vi "Mover4_Control_Forward_Kinematics_Stream_Connection.vi"() -> ()   [LabVIEW 2015]
uses:
  <vilib>/silver_ctls/ArrayMatrixCluster/Real Matrix NI_Silver.ctl
  <vilib>/Utility/miscctls.llb/LVRGBAColorTypeDef.ctl
  <vilib>/robotics/Kinematics/Robot/Forward Kinematics (Point).vi
  <vilib>/robotics/Kinematics/NI_Kinematics.lvlib
  <vilib>/robotics/Kinematics/Plotting/NI_Robotics_3DKinematics.lvlib
panel:
  out "Motor positions (degree)":T1(array[cluster]) {"Error Code (bits)" format="%b"}
  out "End effector transform":T2 format="%#_3g"
  in  "Reset To Zero?":bool
  out "Simulation":refnum<vi>(3d-picture)
  in  "Angles (degree)":dbl[](array[numeric])
  in  "Target IP Address":string="172.22.11.2"
  in  "Stop":bool
  # "In the last column you can see the end effector coordinates (according\nto the theory). This way, you can verify if the real robot reaches this position\ncorrectly."
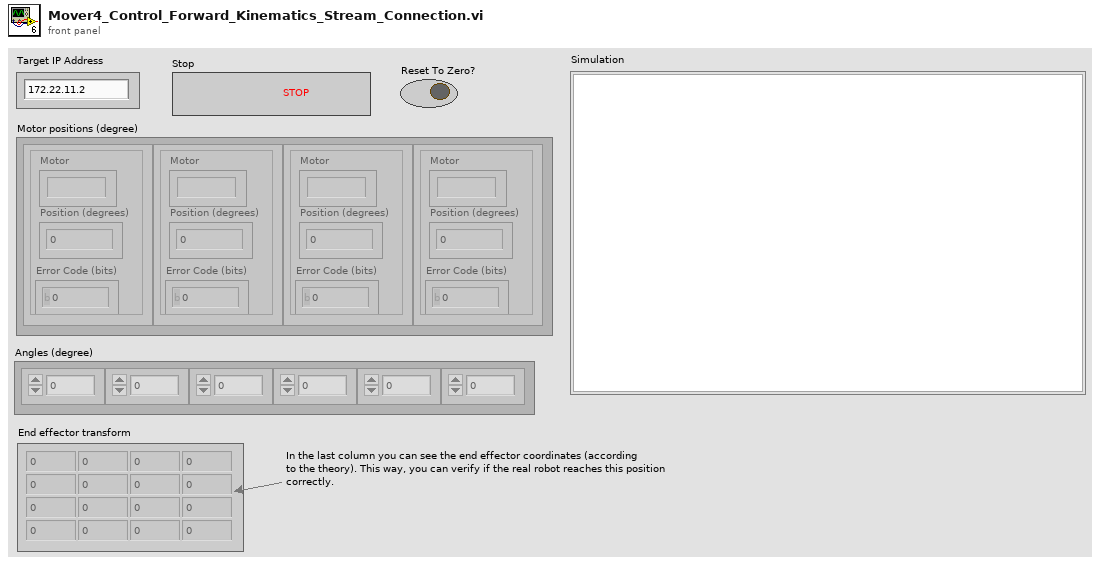
[diagram p1: front panel]
types:
  T1 = cluster{"Position (degrees)":i32, "Error Code (bits)":u8, "Motor":string}[]
  T2 = typedef "Real Matrix NI_Silver.ctl" = dbl[][]
  T3 = typedef "LVRGBAColorTypeDef.ctl" = cluster{"Red":sgl, "Green":sgl, "Blue":sgl, "Alpha":sgl}
  T4 = cluster{"Desired Position":u16, "Enable?":bool, "Reset?":bool}[]
  T5 = cluster{"ID":u8, "Position":u16, "Error Code":u8}[]
  T6 = cluster{"Read Access":enum8{"Allowed", "Required", "None"}, "Write Access":enum8{"Allowed", "Required", "None"}}
  T7 = typedef "NI_Matrix.lvlib/RealMatrix.ctl" = dbl[][]
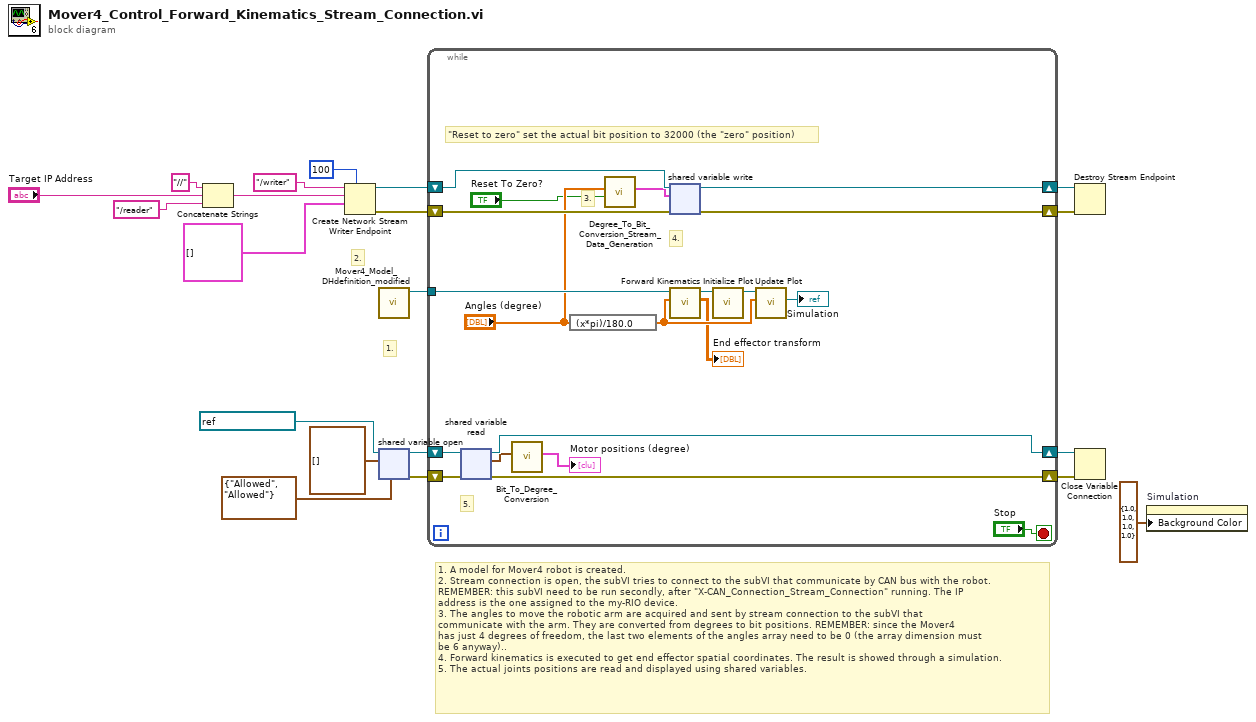
[diagram p0: block diagram]
diagram:
  # "2."
  # "1."
  # "1. A model for Mover4 robot is created.\n2. Stream connection is open, the subVI tries to connect to the subVI that communicate by CAN bus with the robot. \nREMEMBER: this subVI need to be run secondly, after \"X-CAN_Connection_Stream_Connection\" running. The IP\naddress is the one assigned to the my-RIO device. \n3. The angles to move the robotic arm are acquired and sent by stream connection to the subVI that \ncommunicate with the arm. They are converted from degrees to bit positions. REMEMBER: since the Mover4\nhas just 4 degrees of freedom, the last two elements of the angles array need to be 0 (the array dimension must\nbe 6 anyway)..\n4. Forward kinematics is executed to get end effector spatial coordinates. The result is showed through a simulation.\n5. The actual joints positions are read and displayed using shared variables."
  n1 = Concatenate Strings("//", "Target IP Address", "/reader") -> (w13:string)
  n2 = Create Network Stream Writer Endpoint(7:100 ("writer buffer size"), 9:T4 [] ("Commands 2"), 10:w13, 11:"/writer" ("reader name")) -> (0:w6:errorcluster, 3:w7:refnum<k21>)  [unwired: 3 in]
  n3 = call "Mover4_Model_DHdefinition_modified.vi"() -> ("serial arm out"=w2:refnum<class "NI_Robotics_6R Type 1 Serial Arm Class.lvclass">)  [unwired: 10 in, 1 out]
  n4 = shared-variable-open(refnum<k21> "ni.var.psp://stratom-myrio/Shared_Variables/New position" ("shared variable refnum in"), T5 [] ("New position 2"), T6 {"Read Access"=enum."Allowed", "Write Access"=enum."Allowed"} ("access")) -> (w20:refnum<k21>, w19:errorcluster)  [unwired: 1 in]
  n5 = while {
    shift-right: [w38] -> w16
    shift-left: w20 -> [w40]
    shift-right: [w37] -> w15
    shift-left: w19 -> [w39]
    shift-right: [w33] -> w5
    shift-left: w7 -> [w35]
    shift-right: [w32] -> w4
    shift-left: w6 -> [w34]
    tunnel: w2 -> [w31]
    stop <- "Stop" stop-if-true
    # "\"Reset to zero\" set the actual bit position to 32000 (the \"zero\" position)"
    # "5."
    # "4."
    # "3."
    n6 = shared-variable-read(w40, w39) -> (w38:refnum<k21>, w37:errorcluster, w22:T5)  [unwired: 1 out]
    n7 = call "Bit_To_Degree_Conversion.vi"("Actual joints positions"=w22) -> ("Motor positions (degree)"=→"Motor positions (degree)":T1)  [unwired: 10 in]
    n8 = expression code="(x*pi)/180.0"("Angles (degree)") -> (w27:dbl[])
    n9 = call "Degree_To_Bit_Conversion_Stream_Data_Generation.vi"("Reset To Zero?"="Reset To Zero?", "Degree"="Angles (degree)") -> ("Commands"=w25:T4)  [unwired: 9 in]
    n10 = shared-variable-write(w35, w34, w25) -> (w33:refnum<k21>, w32:errorcluster)  [unwired: 1 in, 1 out]
    n11 = call-poly <vilib>:"Forward Kinematics.vi"("joint positions"=w27, "serial arm in"=w31) -> ("end effector transform"=→"End effector transform":T7, "serial arm out"=w30:refnum<class "NI_Robotics_6R Type 1 Serial Arm Class.lvclass">)  [unwired: 7 in, 1 out]
    n12 = call <vilib>:"Initialize Plot.vi"("serial arm in"=w30) -> ("serial arm out"=w29:refnum<class "NI_Robotics_6R Type 1 Serial Arm Class.lvclass">)  [unwired: 9 in, 1 out]
    n13 = call <vilib>:"Update Plot.vi"("joint positions"=w27, "serial arm in"=w29) -> ("serial arm scene"=→"Simulation":refnum<vi>)  [unwired: 7 in, 2 out]
  }
  n14 = Destroy Stream Endpoint(8:w4, 11:w5) -> ()  [unwired: 1 out]
  n15 = Close Variable Connection(8:w15, 11:w16) -> ()  [unwired: 1 out]
  n16 = property on="Simulation" class="SceneGraphDisp (strict)"("Background Color"=T3 {"Red"=1.0, "Green"=1.0, "Blue"=1.0, "Alpha"=1.0}) -> ()  [unwired: 2 in, 2 out]
